vi "Stepper_Final.vi"() -> ()   [LabVIEW 2018]
uses:
  <vilib>/LabVIEW Interface for Arduino/Type Defs/Board Type.ctl
  <vilib>/LabVIEW Interface for Arduino/Type Defs/Connection Type.ctl
  <vilib>/LabVIEW Interface for Arduino/LabVIEW Interface for Arduino.lvlib
panel:
  out "# steps moved":i32
  in  "OK Button":bool
  in  "?":i8(slide) step=2 scale=0.0..2.0
  in  "MOTION":bool
  out "stop motion":bool
  out "Moving?":bool
  in  "Stop":bool
  in  "Arbitray Movement":bool
  in  "Step size":i16
  out "Error":errorcluster
  in  "Total translation distance(in mm)":i16
  out "Steps Remaining?":bool
  out "Iteration #":i32
  in  "Baud Rate":u32=115200
  out "Step Angle":dbl
  in  "Step Size":i16
  out "Steps Remaining?":bool
  in  "Set Speed (Steps/s)":i16=1200 min=0 max=3000 step=50
  in  "Steps for 1 rotation(1600steps)":i16
  in  "Board Type (Uno)":T1
  in  "VISA resource":refnum<visa-resource-name>
  # "For Rotational motion"
  # "For Translational Motion"
  # "For Translational motion"
  # "OFF"
  # "ON"
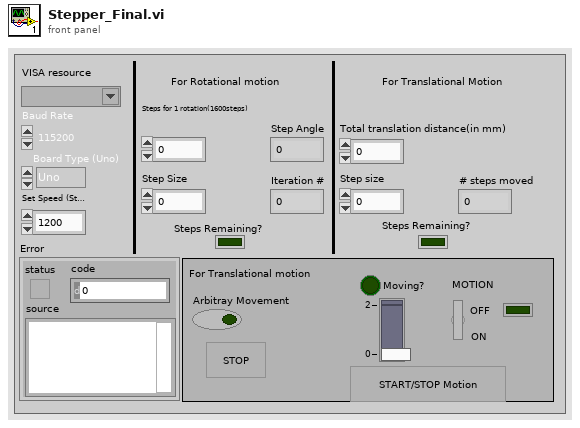
[diagram p1: front panel]
types:
  T1 = typedef "LabVIEW Interface for Arduino.lvlib/Board Type.ctl" = enum16{"Uno", "Dimuelanove w/Atmega 328", "Mega 2560"}
  T2 = typedef "LabVIEW Interface for Arduino.lvlib/Connection Type.ctl" = enum8{"USB / Serial", "XBEE", "BlueSmirf (Bluetooth)"}
  T3 = typedef "LabVIEW Interface for Arduino.lvlib/Arduino Resource.ctl" = cluster{"VISA resource":refnum<visa-resource-name>, "Board Type":T1, "Connection Type":enum8{"USB / Serial"}, "Bytes Per Packet (15)":u8}
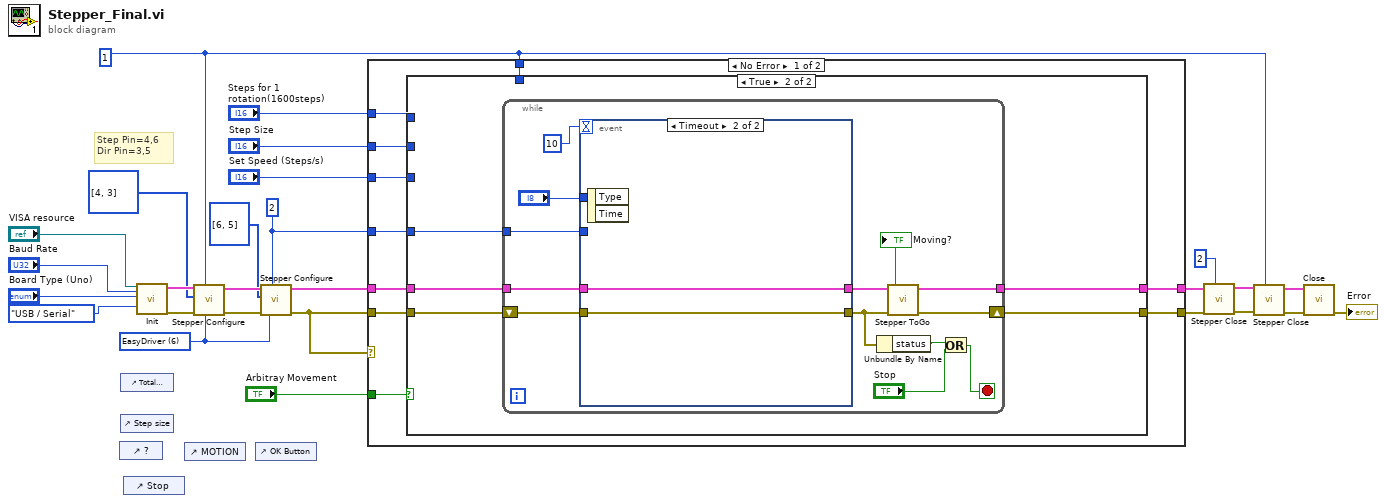
[diagram p0: block diagram]
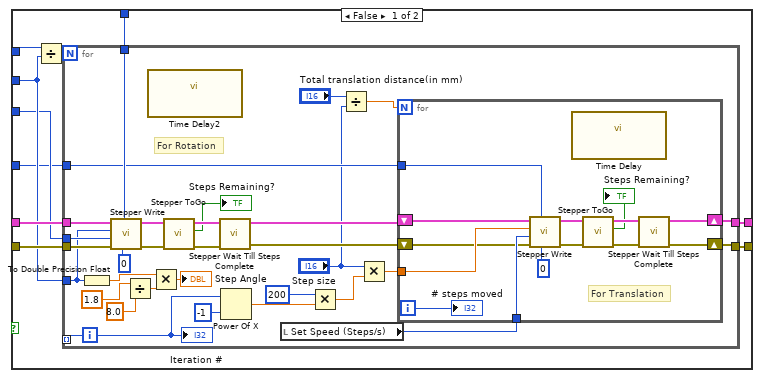
[diagram p2: hidden frame]
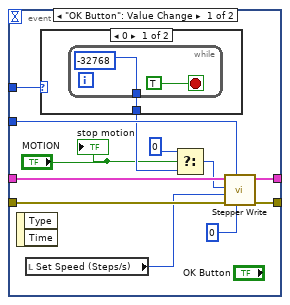
[diagram p3: hidden frame]
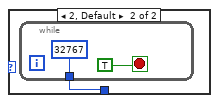
[diagram p4: hidden frame]
diagram:
  w2 = u8 2 ("Stepper #")
  w5 = u8 1 ("Stepper #")
  w3 = u8 6 items=["2 Wire (Pulse & Direction)"=1, "2 Wire"=2, "4 Wire"=4, "EasyDriver"=6, "AF Motor Shield (Stepper 1 & 2 Only)"=5] ("Control Method")
  # "Step Pin=4,6\nDir Pin=3,5"
  n1 = control-ref of="?"() -> ()  [unwired: 1 out]
  n2 = control-ref of="Total translation distance(in mm)"() -> ()  [unwired: 1 out]
  n3 = control-ref of="Step size"() -> ()  [unwired: 1 out]
  n4 = control-ref of="Stop"() -> ()  [unwired: 1 out]
  n5 = call <vilib>:"Init.vi"("VISA resource"="VISA resource", "Baud Rate (115200)"="Baud Rate", "Board Type (Uno)"="Board Type (Uno)", "Connection Type (USB/Serial)"=Connection_Type."USB / Serial") -> ("Arduino Resource"=w24:T3, "error out"=w23:errorcluster)  [unwired: 14 in]
  n6 = control-ref of="MOTION"() -> ()  [unwired: 1 out]
  n7 = call <vilib>:"Stepper Configure.vi"("Control Method"=w3, "Stepper #"=w5, "error in"=w23, "Stepper Pins"=u8[] [4, 3], "Arduino Resource"=w24) -> ("error out"=w7:errorcluster, "Arduino Resource Out"=w9:T3)  [unwired: 5 in]
  n8 = control-ref of="OK Button"() -> ()  [unwired: 1 out]
  n9 = call <vilib>:"Stepper Configure.vi"("Control Method"=w3, "Stepper #"=w2, "error in"=w7, "Stepper Pins"=u8[] [6, 5], "Arduino Resource"=w9) -> ("error out"=w6:errorcluster, "Arduino Resource Out"=w8:T3)  [unwired: 5 in]
  n10 = case shown="No Error" w6 {
    tunnel: [w30 w132] -> w15
    tunnel: [w37 w131] -> w14
    tunnel: w6 -> [w36 w132]
    tunnel: w8 -> [w35 w131]
    tunnel: "Step Size" -> [w34 _]
    tunnel: "Steps for 1 rotation(1600steps)" -> [w33 _]
    tunnel: "Set Speed (Steps/s)" -> [w32 _]
    tunnel: w5 -> [w31 _]
    tunnel: w2 -> [w29 _]
    tunnel: "Arbitray Movement" -> [w28 _]
    frame No Error {
      n11 = case shown="True" w28 {
        tunnel: [w46 w97] -> w37
        tunnel: w36 -> [w45 w94]
        tunnel: w35 -> [w44 w95]
        tunnel: w34 -> [w42 _]
        tunnel: w33 -> [w41 _]
        tunnel: w32 -> [w40 _]
        tunnel: w31 -> [w39 _]
        tunnel: [w47 w96] -> w30
        tunnel: w29 -> [w38 w93]
        frame False {
          n12 = Divide(x=w41, y=w42) -> (x/y=w43:dbl)
          n13 = for {
            N: w43 -> [_]
            tunnel: [w65] -> w47
            tunnel: [w66] -> w46
            tunnel: w45 -> [w75]
            tunnel: w40 -> [w74]
            tunnel: w44 -> [w73]
            tunnel: [w50] -> _ mode=indexing
            tunnel: w42 -> [w68]
            tunnel: w39 -> [w61]
            tunnel: w38 -> [w60]
            i -> [w50]
            # "For Rotation"
            n14 = To Double Precision Float(number=w68) -> (double precision float=w69:dbl)
            n15 = call <vilib>:"Stepper Write.vi"("Set Acceleration (0 to disable)"=i16 0 ("Acceleration"), "Stepper #"=w61, "error in"=w75, "Set Speed (Steps per Second)"=w74, "# of Steps to Move"=w68, "Arduino Resource"=w73) -> ("error out"=w72:errorcluster, "Arduino Resource Out"=w71:T3)  [unwired: 4 in]
            n16 = Divide(x=1.8 ("y"), y=8.0) -> (x/y=w55:dbl)
            n17 = call "Time Delay2"() -> ()  [unwired: 11 in, 1 out]
            n18 = Multiply(x=w69, y=w55) -> (x*y=→"Step Angle":dbl)
            n19 = call <vilib>:"Stepper ToGo.vi"("error in"=w72, "Arduino Resource"=w71) -> ("error out"=w78:errorcluster, "Steps Remaining?"=→"Steps Remaining?":bool, "Arduino Resource Out"=w77:T3)  [unwired: 6 in, 1 out]
            n20 = call <vilib>:"Stepper Wait Till Steps Complete.vi"("error in"=w78, "Arduino Resource In"=w77) -> ("error out"=w67:errorcluster, "Arduino Resource Out"=w64:T3)  [unwired: 8 in]
            n21 = Power Of X(1:-1 ("x"), 2:w50) -> (0:w51:dbl)
            n22 = local read "Set Speed (Steps/s)"() -> (w63:i16)
            n23 = Multiply(x=i16 200 ("y"), y=w51) -> (x*y=w49:dbl)
            n24 = Divide(x="Total translation distance(in mm)", y="Step size") -> (x/y=w53:dbl)
            n25 = Multiply(x="Step size", y=w49) -> (x*y=w57:dbl)
            n26 = for {
              N: w53 -> [_]
              shift-right: [w87] -> w66
              shift-left: w64 -> [w83]
              shift-right: [w86] -> w65
              shift-left: w67 -> [w82]
              tunnel: w57 -> [w85]
              tunnel: w63 -> [w84]
              tunnel: w60 -> [w79]
              i -> [w80]
              # "For Translation"
              n27 = call <vilib>:"Stepper Write.vi"("Set Acceleration (0 to disable)"=i16 0, "Stepper #"=w79, "error in"=w82, "Set Speed (Steps per Second)"=w84, "# of Steps to Move"=w85, "Arduino Resource"=w83) -> ("error out"=w89:errorcluster, "Arduino Resource Out"=w88:T3)  [unwired: 4 in]
              n28 = call "Time Delay"() -> ()  [unwired: 11 in, 1 out]
              n29 = call <vilib>:"Stepper ToGo.vi"("error in"=w89, "Arduino Resource"=w88) -> ("error out"=w92:errorcluster, "Steps Remaining?"=→"Steps Remaining?":bool, "Arduino Resource Out"=w91:T3)  [unwired: 6 in, 1 out]
              n30 = call <vilib>:"Stepper Wait Till Steps Complete.vi"("error in"=w92, "Arduino Resource In"=w91) -> ("error out"=w86:errorcluster, "Arduino Resource Out"=w87:T3)  [unwired: 8 in]
              "# steps moved" <- w80
            }
            "Iteration #" <- w50
          }
        }
        frame True {
          n31 = while {
            shift-right: [w102] -> w96
            shift-left: w94 -> [w110]
            tunnel: [w101] -> w97
            tunnel: w95 -> [w100]
            tunnel: w93 -> [w99]
            stop <- w108 stop-if-true
            n32 = event shown="[1] Timeout" {
              selector: _ -> [_ _]
              dyn-events: _ -> [_ _]
              timeout: 10 -> [_ _]
              tunnel: w110 -> [w121 w129]
              tunnel: w100 -> [w119 w130]
              tunnel: [w120 w130] -> w106
              tunnel: [w122 w129] -> w104
              tunnel: w99 -> [w115 _]
              tunnel: "?" -> [w113 _]
              event "OK Button": Value Change {
                n33 = event-data() -> ()  [unwired: 1 in, 2 out]
                n34 = local read "Set Speed (Steps/s)"() -> (w114:i16)
                n35 = case shown="0" w113 {
                  tunnel: [w123 w126] -> w112
                  frame 0 {
                    n36 = while {
                      tunnel: [i16 -32768 ("# of Steps to Move")] -> w123
                      stop <- TRUE ("Stop Reverse movement") stop-if-true
                    }
                  }
                  frame 2, Default {
                    n37 = while {
                      tunnel: [i16 32767 ("# of Steps to Move")] -> w126
                      stop <- TRUE ("Stop Forward movement") stop-if-true
                    }
                  }
                }
                n38 = Select(t=0, s="MOTION", f=w112) -> (s? t:f=w116:i32)
                n39 = call <vilib>:"Stepper Write.vi"("Set Acceleration (0 to disable)"=i16 0 ("Set acceleration"), "Stepper #"=w115, "error in"=w121, "Set Speed (Steps per Second)"=w114, "# of Steps to Move"=w116, "Arduino Resource"=w119) -> ("error out"=w122:errorcluster, "Arduino Resource Out"=w120:T3)  [unwired: 4 in]
                "stop motion" <- "MOTION"
              }
              event Timeout {
                n40 = event-data() -> ()  [unwired: 1 in, 2 out]
              }
            }
            n41 = Unbundle By Name(w104) -> ("status"=w107:bool)
            n42 = call <vilib>:"Stepper ToGo.vi"("error in"=w104, "Arduino Resource"=w106) -> ("error out"=w102:errorcluster, "Steps Remaining?"=→"Moving?":bool, "Arduino Resource Out"=w101:T3)  [unwired: 6 in, 1 out]
            n43 = Or(x=w107, y="Stop") -> (x .or. y?=w108:bool)
          }
        }
      }
    }
    frame Error {
    }
  }
  n44 = call <vilib>:"Stepper Close.vi"("Stepper #"=u8 2, "error in"=w15, "Arduino Resource"=w14) -> ("error out"=w16:errorcluster, "Arduino Resource Out"=w17:T3)  [unwired: 7 in]
  n45 = call <vilib>:"Stepper Close.vi"("Stepper #"=w5, "error in"=w16, "Arduino Resource"=w17) -> ("error out"=w20:errorcluster, "Arduino Resource Out"=w21:T3)  [unwired: 7 in]
  n46 = call <vilib>:"Close.vi"("Arduino Resource"=w21, "error in"=w20) -> ("error out"=→"Error":errorcluster)  [unwired: 13 in]
